vi "IniState.vi"(8 "error in (no error)":errorcluster, 11 "delta_t":dbl) -> (0 "error out":errorcluster, 1 "params":dbl[](array[numeric]), 2 "Pk":dbl[][](array[numeric]), 3 "xk":dbl[](array[numeric]))   [LabVIEW 2014, in "AppPlugins.lvlib" / "ModelValidationPlugin.lvclass"]
uses:
  ModelValidationPlugin.lvclass
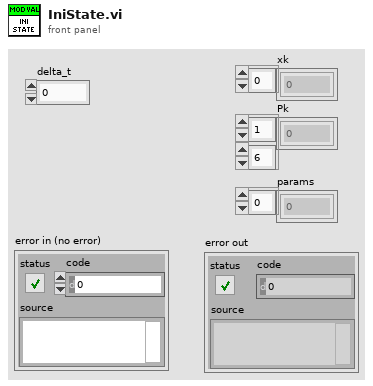
[diagram p1: front panel]
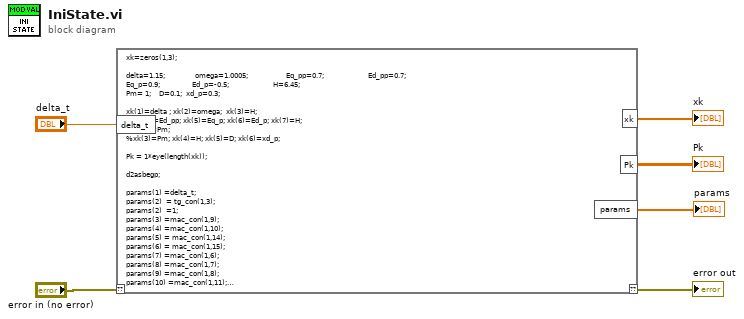
[diagram p0: block diagram]
diagram:
  n1 = script code="xk=zeros(1,3);\n\ndelta=1.15;               omega=1.0005;                   Eq_pp=0.7;                      Ed_pp=0.7;\nEq_p=0.9;                Ed_p=-0.5;                      H=6.45; \nPm= 1;    D=0.1;  xd_p=0.3;\n\nxk(1)=delta ; xk(2)=omega;  xk(3)=H; \n% xk(4)=Ed_pp; xk(5)=Eq_p; xk(6)=Ed_p; xk(7)=H;\n%xk(8)=Pm;\n%xk(3)=Pm; xk(4)=H; xk(5)=D; xk(6)=xd_p; \n\nPk = 1*eye(length(xk));\n\nd2asbegp;\n\nparams(1) =delta_t;\nparams(2)  = tg_con(1,3);\nparams(2)  =1;\nparams(3) =mac_con(1,9);\nparams(4) =mac_con(1,10);\nparams(5) = mac_con(1,14);\nparams(6) = mac_con(1,15);\nparams(7) =mac_con(1,6);\nparams(8) =mac_con(1,7);\nparams(9) =mac_con(1,8);\nparams(10) =mac_con(1,11);\nparams(11) =mac_con(1,12);\nparams(12) =mac_con(1,13);\nparams(13) = 0;\nparams(14) = 1;\nparams(15) = 1; \nparams(16) = mac_con(1,17);"("??"="error in (no error)", "delta_t"="delta_t") -> ("??"=→"error out":errorcluster, "xk"=→"xk":dbl[], "Pk"=→"Pk":dbl[][], "params"=→"params":dbl[])
